vi "Save_image.vi"(0 "Path":string, 1 "remaining elements":T1[](array[typedef])) -> (7 "Number of saved images":i32, 10 "error out":errorcluster)   [LabVIEW 2021]
uses:
  camera_data_cluster.ctl
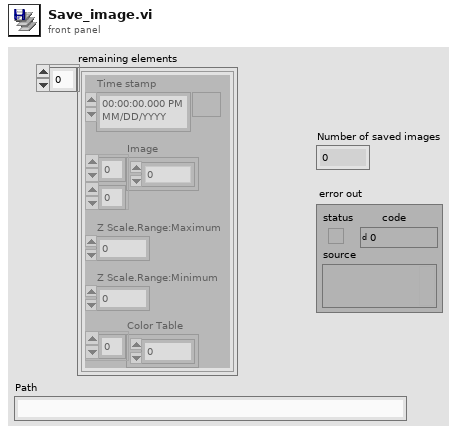
[diagram p1: front panel]
types:
  T1 = typedef "camera_data_cluster.ctl" = cluster{"Time stamp":timestamp, "Image":u8[][], "Z Scale.Range:Maximum":dbl, "Z Scale.Range:Minimum":dbl, "Color Table":u32[]}
  T2 = typedef "imagedata.ctl" = cluster{"image type":i32, "image depth":i32, "image":u8[], "mask":u8[], "colors":u32[], "Rectangle":cluster{"left":i16, "top":i16, "right":i16, "bottom":i16}}
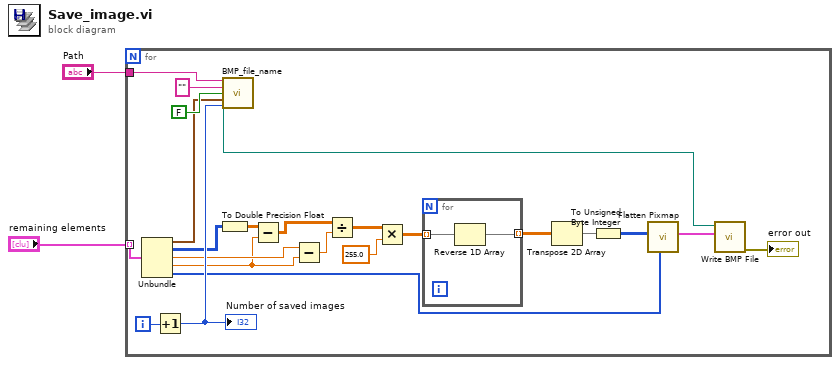
[diagram p0: block diagram]
diagram:
  n1 = for {
    tunnel: "remaining elements" -> [w25] mode=indexing
    tunnel: "Path" -> [w18]
    i -> [w24]
    n2 = Unbundle(w25) -> ("Time stamp"=w20:timestamp, "Image"=w8:u8[][], "Z Scale.Range:Maximum"=w15:dbl, "Z Scale.Range:Minimum"=w14:dbl, "Color Table"=w3:u32[])
    n3 = Increment(x=w24) -> (x+1=w19:i32)
    "Number of saved images" <- w19
    n4 = To Double Precision Float(number=w8) -> (double precision float=w9:dbl[][])
    n5 = call "BMP_file_name.vi"("Path_to_folder_to_save_bmp_imgs"=w18, "Additional_text_information"="", "Laser_status_ON_OFF"=FALSE, "time stamp"=w20, "Image_number"=w19) -> ("file path"=w17:path)  [unwired: 10 in]
    n6 = Subtract(x=w9, y=w14) -> (x-y=w13:dbl[][])
    n7 = Subtract(x=w15, y=w14) -> (x-y=w12:dbl)
    n8 = Divide(x=w13, y=w12) -> (x/y=w11:dbl[][])
    n9 = Multiply(x=w11, y=255.0) -> (x*y=w7:dbl[][])
    n10 = for {
      tunnel: w7 -> [w27] mode=indexing
      tunnel: [w26] -> w6 mode=indexing
      n11 = Reverse 1D Array(array=w27) -> (reversed array=w26:dbl[])
    }
    n12 = Transpose 2D Array(2D array=w6) -> (transposed array=w5:dbl[][])
    n13 = To Unsigned Byte Integer(number=w5) -> (unsigned 8bit integer=w4:u8[][])
    n14 = call <vilib>:"Flatten Pixmap.vi"("colors"=w3, "8-bit pixmap"=w4) -> ("image data"=w16:T2)  [unwired: 9 in]
    n15 = call <vilib>:"Write BMP File.vi"("image data"=w16, "path to BMP file"=w17) -> ("error out"=→"error out":errorcluster)  [unwired: 8 in, 1 out]
  }
